vi "ZMC Search Eth.vi"(8 "error in (no error)":errorcluster caption="错误输入（无错误）", 9 "uims":u32, 10 "addrbufflength":u32, 11 "ipaddrlist":string) -> (0 "error out":errorcluster caption="错误输出", 2 "function return":i32, 3 "ipaddrlist out":string)   [LabVIEW 2015, in "zauxdll.lvlib"]
doc: "int32 __stdcall ZMC_SearchEth(char *ipaddrlist, uint32 addrbufflength, uint32 uims);"
uses:
  zauxdll.lvlib
  zmotion.dll
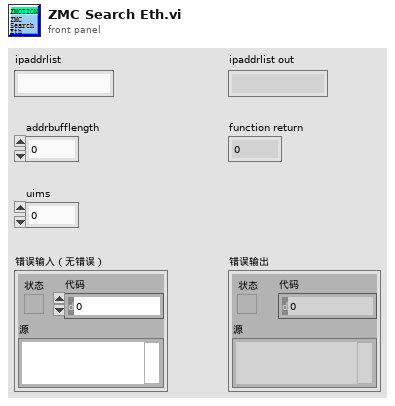
[diagram p1: front panel]
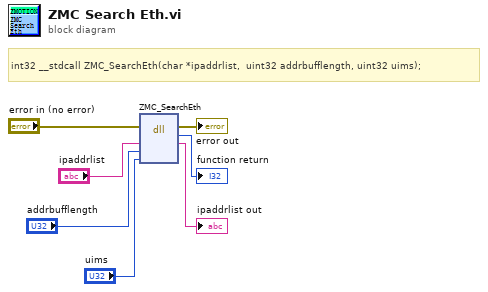
[diagram p0: block diagram]
diagram:
  # "int32 __stdcall ZMC_SearchEth(char *ipaddrlist,  uint32 addrbufflength, uint32 uims);"
  n1 = dll-call lib="C:/Users/VIC/Desktop/GOGORO_SA/system/LLB/zmotion/zaux/zmotion.*" fn="ZMC_SearchEth"(error in="error in (no error)", "ipaddrlist"="ipaddrlist", "addrbufflength"="addrbufflength", "uims"="uims") -> (error out=→"error out":errorcluster, →"function return":i32, "ipaddrlist"=→"ipaddrlist out":string)  [unwired: 4 in, 1 out]
